vi "Calculate Gains.vi"(1 "DSA Averages":T5, 2 "WT1800 Averages":T3 {"Vrms" format="%.3f"; "Irms" format="%.3f"; "Power" format="%.3f"; "Vpkpk" format="%.3f"; "Ipkpk" format="%.3f"}, 11 "error in":errorcluster, 12 "Error or Abort":bool, 13 "Settings Cluster":T7={"Supply Voltage [Vdc]"=0.0, "Max Supply Current [Idc]"=0.0, "Settling Delay"=0.0, "Temp Criteria"=0.0, "Voltage Steps [Vrms]"=[], "User Notes"="", "Config Wave File Path"=path "", "Config Voltage [Vrms]"=0.0, "Channel Configuration List"={"Channel Configuration Cluster"={"Input"=enum."---", "Enable"=FALSE, "User Notes"="", "Voltage Range"=15.0, "Current Range"=2.5}, "Channel Configuration Cluster 2"={"Input"=enum."---", "Enable"=FALSE, "User Notes"="", "Voltage Range"=15.0, "Current Range"=2.5}, "Channel Configuration Cluster 3"={"Input"=enum."---", "Enable"=FALSE, "User Notes"="", "Voltage Range"=15.0, "Current Range"=2.5}, "Channel Configuration Cluster 4"={"Input"=enum."---", "Enable"=FALSE, "User Notes"="", "Voltage Range"=15.0, "Current Range"=2.5}, "Channel Configuration Cluster 5"={"Input"=enum."---", "Enable"=FALSE, "User Notes"="", "Voltage Range"=15.0, "Current Range"=2.5}, "Channel Configuration Cluster 6"={"Input"=enum."---", "Enable"=FALSE, "User Notes"="", "Voltage Range"=15.0, "Current Range"=2.5}, "Channel Configuration Cluster 7"={"Input"=enum."---", "Enable"=FALSE, "User Notes"="", "Voltage Range"=15.0, "Current Range"=2.5}, "Channel Configuration Cluster 8"={"Input"=enum."---", "Enable"=FALSE, "User Notes"="", "Voltage Range"=15.0, "Current Range"=2.5}, "Channel Configuration Cluster 9"={"Input"=enum."---", "Enable"=FALSE, "User Notes"="", "Voltage Range"=15.0, "Current Range"=2.5}, "Channel Configuration Cluster 10"={"Input"=enum."---", "Enable"=FALSE, "User Notes"="", "Voltage Range"=15.0, "Current Range"=25.0}, "Channel Configuration Cluster 11"={"Input"=enum."---", "Enable"=FALSE, "User Notes"="", "Voltage Range"=15.0, "Current Range"=25.0}, "Channel Configuration Cluster 12"={"Input"=enum."---", "Enable"=FALSE, "User Notes"="", "Voltage Range"=15.0, "Current Range"=25.0}, "Channel Configuration Cluster 13"={"Input"=enum."---", "Enable"=FALSE, "User Notes"="", "Voltage Range"=15.0, "Current Range"=25.0}, "Channel Configuration Cluster 14"={"Input"=enum."---", "Enable"=FALSE, "User Notes"="", "Voltage Range"=15.0, "Current Range"=25.0}, "Channel Configuration Cluster 15"={"Input"=enum."---", "Enable"=FALSE, "User Notes"="", "Voltage Range"=15.0, "Current Range"=25.0}, "Channel Configuration Cluster 16"={"Input"=enum."---", "Enable"=FALSE, "User Notes"="", "Voltage Range"=15.0, "Current Range"=25.0}, "Channel Configuration Cluster 17"={"Input"=enum."---", "Enable"=FALSE, "User Notes"="", "Voltage Range"=15.0, "Current Range"=25.0}}, "User Gains"={"Gain 1"=0.0, "Gain 2"=0.0, "Gain 3"=0.0, "Gain 4"=0.0, "Gain 5"=0.0, "Gain 6"=0.0}, "Gains"={"Gain 1"=0.0, "Gain 2"=0.0, "Gain 3"=0.0, "Gain 4"=0.0, "Gain 5"=0.0, "Gain 6"=0.0}, "Gain Array"={"Gain 1"=0.0, "Gain 2"=0.0, "Gain 3"=0.0, "Gain 4"=0.0, "Gain 5"=0.0, "Gain 6"=0.0, "Gain 7"=0.0, "Gain 8"=0.0, "Gain 9"=0.0, "Gain 10"=0.0, "Gain 11"=0.0, "Gain 12"=0.0, "Gain 13"=0.0, "Gain 14"=0.0, "Gain 15"=0.0, "Gain 16"=0.0, "Gain 17"=0.0}, "Wave File Path 1"=path "", "Wave File Path 2"=path "", "Wave File Path 3"=path "", "Wave File Path 4"=path "", "Range"=FALSE, "CF"=FALSE} {"Gain Array"."Gain 17" format="%.2f"; "Gain Array"."Gain 16" format="%.2f"; "Gain Array"."Gain 15" format="%.2f"; "Gain Array"."Gain 14" format="%.2f"; "Gain Array"."Gain 13" format="%.2f"; "Gain Array"."Gain 12" format="%.2f"; "Gain Array"."Gain 11" format="%.2f"; "Gain Array"."Gain 10" format="%.2f"; "Gain Array"."Gain 9" format="%.2f"; "Gain Array"."Gain 8" format="%.2f"; "Gain Array"."Gain 7" format="%.2f"; "Gain Array"."Gain 6" format="%.2f"; "Gain Array"."Gain 5" format="%.2f"; "Gain Array"."Gain 4" format="%.2f"; "Gain Array"."Gain 3" format="%.2f"; "Gain Array"."Gain 2" format="%.2f"; "Gain Array"."Gain 1" format="%.2f"; "Gains"."Gain 6" format="%.2f"; "Gains"."Gain 5" format="%.2f"; "Gains"."Gain 4" format="%.2f"; "Gains"."Gain 3" format="%.2f"; "Gains"."Gain 2" format="%.2f"; "Gains"."Gain 1" format="%.2f"; "User Gains"."Gain 6" format="%.2f"; "User Gains"."Gain 5" format="%.2f"; "User Gains"."Gain 4" format="%.2f"; "User Gains"."Gain 3" format="%.2f"; "User Gains"."Gain 2" format="%.2f"; "User Gains"."Gain 1" format="%.2f"; "Channel Configuration List"."Channel Configuration Cluster 17"."Current Range" items=["1 <500m>"=0.5, "2 <1>"=1.0, "5 <2.5>"=2.5, "10 <5>"=5.0, "20 <10>"=10.0, "50 <25>"=25.0]; "Channel Configuration List"."Channel Configuration Cluster 17"."Voltage Range" items=["1.5 <0.75>"=0.75, "3 <1.5>"=1.5, "6 <3>"=3.0, "10 <5>"=5.0, "15 <7.5>"=7.5, "30 <15>"=15.0, "60 <30>"=30.0, "100 <50>"=50.0, "150 <75>"=75.0, "300 <150>"=150.0, "600 <300>"=300.0, "1000 <500>"=500.0]; "Channel Configuration List"."Channel Configuration Cluster 16"."Current Range" items=["1 <500m>"=0.5, "2 <1>"=1.0, "5 <2.5>"=2.5, "10 <5>"=5.0, "20 <10>"=10.0, "50 <25>"=25.0]; "Channel Configuration List"."Channel Configuration Cluster 16"."Voltage Range" items=["1.5 <0.75>"=0.75, "3 <1.5>"=1.5, "6 <3>"=3.0, "10 <5>"=5.0, "15 <7.5>"=7.5, "30 <15>"=15.0, "60 <30>"=30.0, "100 <50>"=50.0, "150 <75>"=75.0, "300 <150>"=150.0, "600 <300>"=300.0, "1000 <500>"=500.0]; "Channel Configuration List"."Channel Configuration Cluster 15"."Current Range" items=["1 <500m>"=0.5, "2 <1>"=1.0, "5 <2.5>"=2.5, "10 <5>"=5.0, "20 <10>"=10.0, "50 <25>"=25.0]; "Channel Configuration List"."Channel Configuration Cluster 15"."Voltage Range" items=["1.5 <0.75>"=0.75, "3 <1.5>"=1.5, "6 <3>"=3.0, "10 <5>"=5.0, "15 <7.5>"=7.5, "30 <15>"=15.0, "60 <30>"=30.0, "100 <50>"=50.0, "150 <75>"=75.0, "300 <150>"=150.0, "600 <300>"=300.0, "1000 <500>"=500.0]; "Channel Configuration List"."Channel Configuration Cluster 14"."Current Range" items=["1 <500m>"=0.5, "2 <1>"=1.0, "5 <2.5>"=2.5, "10 <5>"=5.0, "20 <10>"=10.0, "50 <25>"=25.0]; "Channel Configuration List"."Channel Configuration Cluster 14"."Voltage Range" items=["1.5 <0.75>"=0.75, "3 <1.5>"=1.5, "6 <3>"=3.0, "10 <5>"=5.0, "15 <7.5>"=7.5, "30 <15>"=15.0, "60 <30>"=30.0, "100 <50>"=50.0, "150 <75>"=75.0, "300 <150>"=150.0, "600 <300>"=300.0, "1000 <500>"=500.0]; "Channel Configuration List"."Channel Configuration Cluster 13"."Current Range" items=["1 <500m>"=0.5, "2 <1>"=1.0, "5 <2.5>"=2.5, "10 <5>"=5.0, "20 <10>"=10.0, "50 <25>"=25.0]; "Channel Configuration List"."Channel Configuration Cluster 13"."Voltage Range" items=["1.5 <0.75>"=0.75, "3 <1.5>"=1.5, "6 <3>"=3.0, "10 <5>"=5.0, "15 <7.5>"=7.5, "30 <15>"=15.0, "60 <30>"=30.0, "100 <50>"=50.0, "150 <75>"=75.0, "300 <150>"=150.0, "600 <300>"=300.0, "1000 <500>"=500.0]; "Channel Configuration List"."Channel Configuration Cluster 12"."Current Range" items=["1 <500m>"=0.5, "2 <1>"=1.0, "5 <2.5>"=2.5, "10 <5>"=5.0, "20 <10>"=10.0, "50 <25>"=25.0]; "Channel Configuration List"."Channel Configuration Cluster 12"."Voltage Range" items=["1.5 <0.75>"=0.75, "3 <1.5>"=1.5, "6 <3>"=3.0, "10 <5>"=5.0, "15 <7.5>"=7.5, "30 <15>"=15.0, "60 <30>"=30.0, "100 <50>"=50.0, "150 <75>"=75.0, "300 <150>"=150.0, "600 <300>"=300.0, "1000 <500>"=500.0]; "Channel Configuration List"."Channel Configuration Cluster 11"."Current Range" items=["1 <500m>"=0.5, "2 <1>"=1.0, "5 <2.5>"=2.5, "10 <5>"=5.0, "20 <10>"=10.0, "50 <25>"=25.0]; "Channel Configuration List"."Channel Configuration Cluster 11"."Voltage Range" items=["1.5 <0.75>"=0.75, "3 <1.5>"=1.5, "6 <3>"=3.0, "10 <5>"=5.0, "15 <7.5>"=7.5, "30 <15>"=15.0, "60 <30>"=30.0, "100 <50>"=50.0, "150 <75>"=75.0, "300 <150>"=150.0, "600 <300>"=300.0, "1000 <500>"=500.0]; "Channel Configuration List"."Channel Configuration Cluster 10"."Current Range" items=["1 <500m>"=0.5, "2 <1>"=1.0, "5 <2.5>"=2.5, "10 <5>"=5.0, "20 <10>"=10.0, "50 <25>"=25.0]; "Channel Configuration List"."Channel Configuration Cluster 10"."Voltage Range" items=["1.5 <0.75>"=0.75, "3 <1.5>"=1.5, "6 <3>"=3.0, "10 <5>"=5.0, "15 <7.5>"=7.5, "30 <15>"=15.0, "60 <30>"=30.0, "100 <50>"=50.0, "150 <75>"=75.0, "300 <150>"=150.0, "600 <300>"=300.0, "1000 <500>"=500.0]; "Channel Configuration List"."Channel Configuration Cluster 9"."Voltage Range" items=["1.5 <0.75>"=0.75, "3 <1.5>"=1.5, "6 <3>"=3.0, "10 <5>"=5.0, "15 <7.5>"=7.5, "30 <15>"=15.0, "60 <30>"=30.0, "100 <50>"=50.0, "150 <75>"=75.0, "300 <150>"=150.0, "600 <300>"=300.0, "1000 <500>"=500.0]; "Channel Configuration List"."Channel Configuration Cluster 9"."Current Range" items=["10m <5m>"=0.005, "20m <10m>"=0.01, "50m <25m>"=0.025, "100m <50m>"=0.05, "200m <100m>"=0.1, "500m <250m>"=0.25, "1 <500m>"=0.5, "2 <1>"=1.0, "5 <2.5>"=2.5]; "Channel Configuration List"."Channel Configuration Cluster 8"."Voltage Range" items=["1.5 <0.75>"=0.75, "3 <1.5>"=1.5, "6 <3>"=3.0, "10 <5>"=5.0, "15 <7.5>"=7.5, "30 <15>"=15.0, "60 <30>"=30.0, "100 <50>"=50.0, "150 <75>"=75.0, "300 <150>"=150.0, "600 <300>"=300.0, "1000 <500>"=500.0]; "Channel Configuration List"."Channel Configuration Cluster 8"."Current Range" items=["10m <5m>"=0.005, "20m <10m>"=0.01, "50m <25m>"=0.025, "100m <50m>"=0.05, "200m <100m>"=0.1, "500m <250m>"=0.25, "1 <500m>"=0.5, "2 <1>"=1.0, "5 <2.5>"=2.5]; "Channel Configuration List"."Channel Configuration Cluster 7"."Voltage Range" items=["1.5 <0.75>"=0.75, "3 <1.5>"=1.5, "6 <3>"=3.0, "10 <5>"=5.0, "15 <7.5>"=7.5, "30 <15>"=15.0, "60 <30>"=30.0, "100 <50>"=50.0, "150 <75>"=75.0, "300 <150>"=150.0, "600 <300>"=300.0, "1000 <500>"=500.0]; "Channel Configuration List"."Channel Configuration Cluster 7"."Current Range" items=["10m <5m>"=0.005, "20m <10m>"=0.01, "50m <25m>"=0.025, "100m <50m>"=0.05, "200m <100m>"=0.1, "500m <250m>"=0.25, "1 <500m>"=0.5, "2 <1>"=1.0, "5 <2.5>"=2.5]; "Channel Configuration List"."Channel Configuration Cluster 6"."Voltage Range" items=["1.5 <0.75>"=0.75, "3 <1.5>"=1.5, "6 <3>"=3.0, "10 <5>"=5.0, "15 <7.5>"=7.5, "30 <15>"=15.0, "60 <30>"=30.0, "100 <50>"=50.0, "150 <75>"=75.0, "300 <150>"=150.0, "600 <300>"=300.0, "1000 <500>"=500.0]; "Channel Configuration List"."Channel Configuration Cluster 6"."Current Range" items=["10m <5m>"=0.005, "20m <10m>"=0.01, "50m <25m>"=0.025, "100m <50m>"=0.05, "200m <100m>"=0.1, "500m <250m>"=0.25, "1 <500m>"=0.5, "2 <1>"=1.0, "5 <2.5>"=2.5]; "Channel Configuration List"."Channel Configuration Cluster 5"."Voltage Range" items=["1.5 <0.75>"=0.75, "3 <1.5>"=1.5, "6 <3>"=3.0, "10 <5>"=5.0, "15 <7.5>"=7.5, "30 <15>"=15.0, "60 <30>"=30.0, "100 <50>"=50.0, "150 <75>"=75.0, "300 <150>"=150.0, "600 <300>"=300.0, "1000 <500>"=500.0]; "Channel Configuration List"."Channel Configuration Cluster 5"."Current Range" items=["10m <5m>"=0.005, "20m <10m>"=0.01, "50m <25m>"=0.025, "100m <50m>"=0.05, "200m <100m>"=0.1, "500m <250m>"=0.25, "1 <500m>"=0.5, "2 <1>"=1.0, "5 <2.5>"=2.5]; "Channel Configuration List"."Channel Configuration Cluster 4"."Voltage Range" items=["1.5 <0.75>"=0.75, "3 <1.5>"=1.5, "6 <3>"=3.0, "10 <5>"=5.0, "15 <7.5>"=7.5, "30 <15>"=15.0, "60 <30>"=30.0, "100 <50>"=50.0, "150 <75>"=75.0, "300 <150>"=150.0, "600 <300>"=300.0, "1000 <500>"=500.0]; "Channel Configuration List"."Channel Configuration Cluster 4"."Current Range" items=["10m <5m>"=0.005, "20m <10m>"=0.01, "50m <25m>"=0.025, "100m <50m>"=0.05, "200m <100m>"=0.1, "500m <250m>"=0.25, "1 <500m>"=0.5, "2 <1>"=1.0, "5 <2.5>"=2.5]; "Channel Configuration List"."Channel Configuration Cluster 3"."Voltage Range" items=["1.5 <0.75>"=0.75, "3 <1.5>"=1.5, "6 <3>"=3.0, "10 <5>"=5.0, "15 <7.5>"=7.5, "30 <15>"=15.0, "60 <30>"=30.0, "100 <50>"=50.0, "150 <75>"=75.0, "300 <150>"=150.0, "600 <300>"=300.0, "1000 <500>"=500.0]; "Channel Configuration List"."Channel Configuration Cluster 3"."Current Range" items=["10m <5m>"=0.005, "20m <10m>"=0.01, "50m <25m>"=0.025, "100m <50m>"=0.05, "200m <100m>"=0.1, "500m <250m>"=0.25, "1 <500m>"=0.5, "2 <1>"=1.0, "5 <2.5>"=2.5]; "Channel Configuration List"."Channel Configuration Cluster 2"."Voltage Range" items=["1.5 <0.75>"=0.75, "3 <1.5>"=1.5, "6 <3>"=3.0, "10 <5>"=5.0, "15 <7.5>"=7.5, "30 <15>"=15.0, "60 <30>"=30.0, "100 <50>"=50.0, "150 <75>"=75.0, "300 <150>"=150.0, "600 <300>"=300.0, "1000 <500>"=500.0]; "Channel Configuration List"."Channel Configuration Cluster 2"."Current Range" items=["10m <5m>"=0.005, "20m <10m>"=0.01, "50m <25m>"=0.025, "100m <50m>"=0.05, "200m <100m>"=0.1, "500m <250m>"=0.25, "1 <500m>"=0.5, "2 <1>"=1.0, "5 <2.5>"=2.5]; "Channel Configuration List"."Channel Configuration Cluster"."Voltage Range" items=["1.5 <0.75>"=0.75, "3 <1.5>"=1.5, "6 <3>"=3.0, "10 <5>"=5.0, "15 <7.5>"=7.5, "30 <15>"=15.0, "60 <30>"=30.0, "100 <50>"=50.0, "150 <75>"=75.0, "300 <150>"=150.0, "600 <300>"=300.0, "1000 <500>"=500.0]; "Channel Configuration List"."Channel Configuration Cluster"."Current Range" items=["10m <5m>"=0.005, "20m <10m>"=0.01, "50m <25m>"=0.025, "100m <50m>"=0.05, "200m <100m>"=0.1, "500m <250m>"=0.25, "1 <500m>"=0.5, "2 <1>"=1.0, "5 <2.5>"=2.5]; "Settling Delay" min=0.0 format="%<%H:%M:%S>t"}) -> (4 "Average Power":sgl[](array[numeric]) format="%.3g", 6 "Gain Averages":T1 {"Gain 6" format="%.2f"; "Gain 5" format="%.2f"; "Gain 4" format="%.2f"; "Gain 3" format="%.2f"; "Gain 2" format="%.2f"; "Gain 1" format="%.2f"}, 8 "Gain Array":T2 {"Gain 17" format="%.2f"; "Gain 16" format="%.2f"; "Gain 15" format="%.2f"; "Gain 14" format="%.2f"; "Gain 13" format="%.2f"; "Gain 12" format="%.2f"; "Gain 11" format="%.2f"; "Gain 10" format="%.2f"; "Gain 9" format="%.2f"; "Gain 8" format="%.2f"; "Gain 7" format="%.2f"; "Gain 6" format="%.2f"; "Gain 5" format="%.2f"; "Gain 4" format="%.2f"; "Gain 3" format="%.2f"; "Gain 2" format="%.2f"; "Gain 1" format="%.2f"}, 14 "Impedances":dbl[](array[numeric]) format="%.3g", 15 "error out":errorcluster)   [LabVIEW 2021]
uses:
  Controls/Settings Control.ctl
  Controls/Channel Configuration List.ctl
  Controls/Channel Configuration Cluster.ctl
  Controls/Channel Configuration Cluster High Current.ctl
  Controls/Gain Averages.ctl
  Controls/Gain Array.ctl
  Controls/WT1800 Measurements.ctl
  Controls/WT1800 Readings.ctl
  Controls/DSA Measurements.ctl
  Controls/DSA Readings.ctl
  <vilib>/Analysis/baseanly.llb/Mean (DBL).vi
  <vilib>/Analysis/NI_AALBase.lvlib
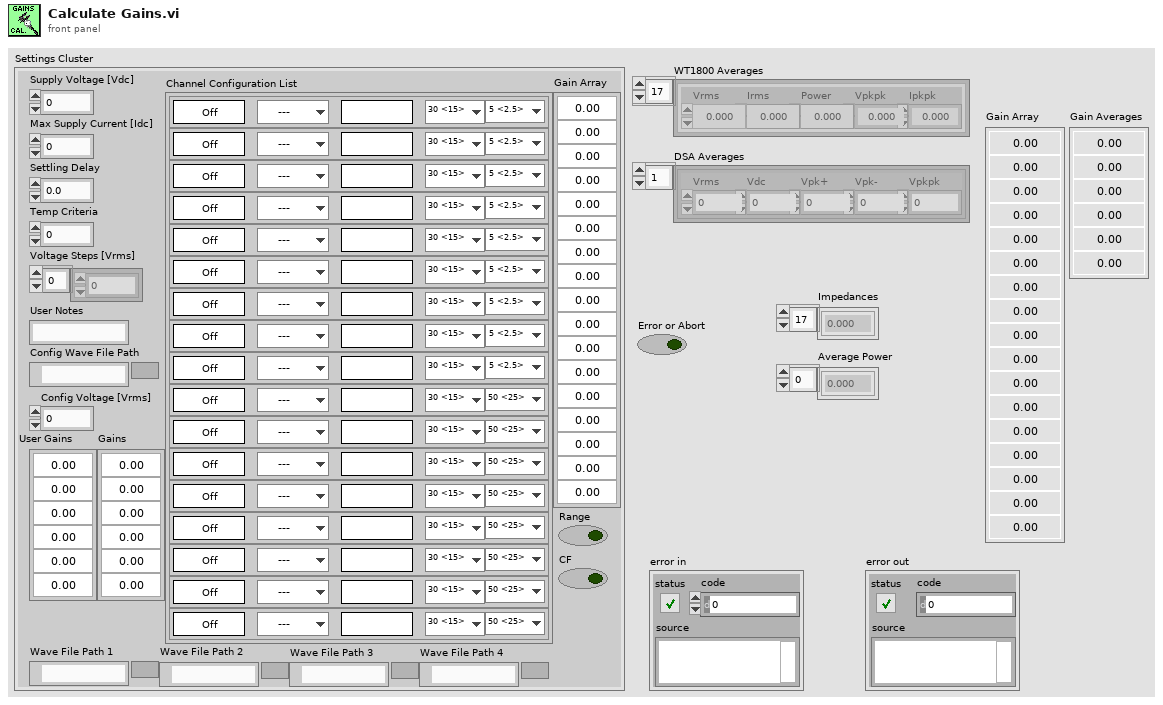
[diagram p1: front panel]
types:
  T1 = typedef "Gain Averages.ctl" = cluster{"Gain 1":dbl, "Gain 2":dbl, "Gain 3":dbl, "Gain 4":dbl, "Gain 5":dbl, "Gain 6":dbl}
  T2 = typedef "Gain Array.ctl" = cluster{"Gain 1":dbl, "Gain 2":dbl, "Gain 3":dbl, "Gain 4":dbl, "Gain 5":dbl, "Gain 6":dbl, "Gain 7":dbl, "Gain 8":dbl, "Gain 9":dbl, "Gain 10":dbl, "Gain 11":dbl, "Gain 12":dbl, "Gain 13":dbl, "Gain 14":dbl, "Gain 15":dbl, "Gain 16":dbl, "Gain 17":dbl}
  T3 = typedef "WT1800 Measurements.ctl" = T4[]
  T4 = typedef "WT1800 Readings.ctl" = cluster{"Vrms":sgl, "Irms":sgl, "Power":sgl, "Vpkpk":sgl, "Ipkpk":sgl}
  T5 = typedef "DSA Measurements.ctl" = T6[]
  T6 = typedef "DSA Readings.ctl" = cluster{"Vrms":sgl, "Vdc":sgl, "Vpk+":sgl, "Vpk-":sgl, "Vpkpk":sgl}
  T7 = typedef "Settings Control.ctl" = cluster{"Supply Voltage [Vdc]":sgl, "Max Supply Current [Idc]":sgl, "Settling Delay":dbl, "Temp Criteria":sgl, "Voltage Steps [Vrms]":sgl[], "User Notes":string, "Config Wave File Path":path, "Config Voltage [Vrms]":sgl, "Channel Configuration List":T8, "User Gains":T1, "Gains":T1, "Gain Array":T2, "Wave File Path 1":path, "Wave File Path 2":path, "Wave File Path 3":path, "Wave File Path 4":path, "Range":bool, "CF":bool}
  T8 = typedef "Channel Configuration List.ctl" = cluster{"Channel Configuration Cluster":T9, "Channel Configuration Cluster 2":T9, "Channel Configuration Cluster 3":T9, "Channel Configuration Cluster 4":T9, "Channel Configuration Cluster 5":T9, "Channel Configuration Cluster 6":T9, "Channel Configuration Cluster 7":T9, "Channel Configuration Cluster 8":T9, "Channel Configuration Cluster 9":T9, "Channel Configuration Cluster 10":T10, "Channel Configuration Cluster 11":T10, "Channel Configuration Cluster 12":T10, "Channel Configuration Cluster 13":T10, "Channel Configuration Cluster 14":T10, "Channel Configuration Cluster 15":T10, "Channel Configuration Cluster 16":T10, "Channel Configuration Cluster 17":T10}
  T9 = typedef "Channel Configuration Cluster.ctl" = cluster{"Input":enum16{"---", "1", "1 AVG", "2", "2 AVG", "3", "3 AVG", "4", "4 AVG"}, "Enable":bool, "User Notes":string, "Voltage Range":dbl, "Current Range":dbl}
  T10 = typedef "Channel Configuration Cluster High Current.ctl" = cluster{"Input":enum16{"---", "1", "1 AVG", "2", "2 AVG", "3", "3 AVG", "4", "4 AVG"}, "Enable":bool, "User Notes":string, "Voltage Range":dbl, "Current Range":dbl}
  T11 = enum16{"---", "1", "1 AVG", "2", "2 AVG", "3", "3 AVG", "4", "4 AVG"}
  T12 = cluster{"[0]":dbl, "[1]":dbl, "[2]":dbl, "[3]":dbl, "[4]":dbl, "[5]":dbl}
  T13 = cluster{"[0]":dbl, "[1]":dbl, "[2]":dbl, "[3]":dbl, "[4]":dbl, "[5]":dbl, "[6]":dbl, "[7]":dbl, "[8]":dbl, "[9]":dbl, "[10]":dbl, "[11]":dbl, "[12]":dbl, "[13]":dbl, "[14]":dbl, "[15]":dbl, "[16]":dbl}
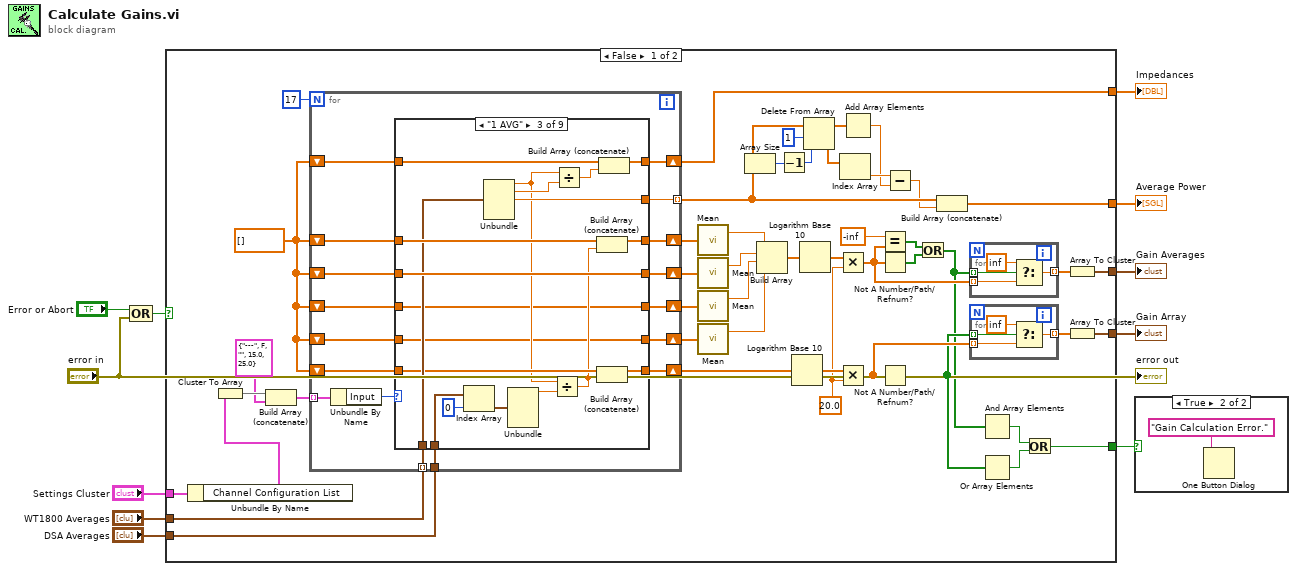
[diagram p0: block diagram]
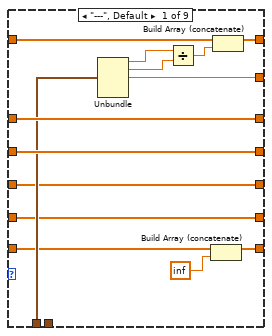
[diagram p3: hidden frame]
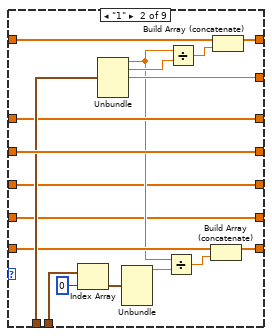
[diagram p4: hidden frame]
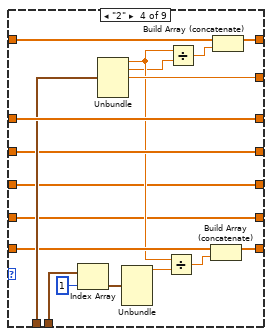
[diagram p5: hidden frame]
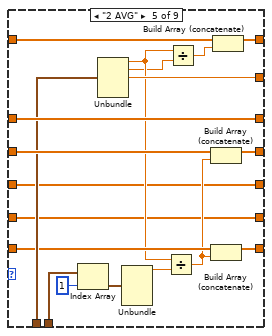
[diagram p6: hidden frame]
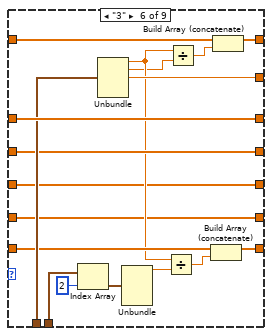
[diagram p7: hidden frame]
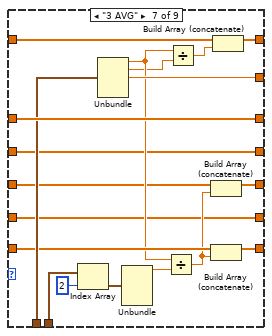
[diagram p8: hidden frame]
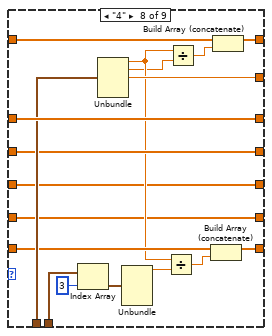
[diagram p9: hidden frame]
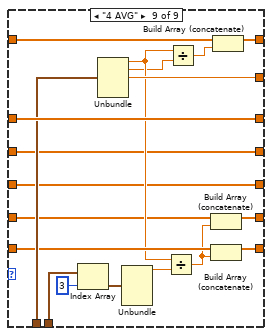
[diagram p10: hidden frame]
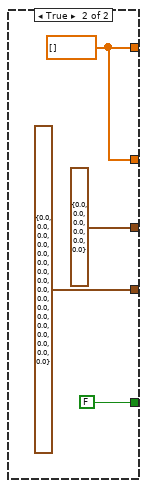
[diagram p11: hidden frame]
diagram:
  n1 = Compound Arithmetic op=OR("Error or Abort", "error in") -> (w4:bool)
  n2 = case shown="False" w4 {
    tunnel: "Settings Cluster" -> [w38 _]
    tunnel: "DSA Averages" -> [w36 _]
    tunnel: "WT1800 Averages" -> [w37 _]
    tunnel: [w35 w249] -> w11
    tunnel: [w56 T2 {"Gain 1"=0.0, "Gain 2"=0.0, "Gain 3"=0.0, "Gain 4"=0.0, "Gain 5"=0.0, "Gain 6"=0.0, "Gain 7"=0.0, "Gain 8"=0.0, "Gain 9"=0.0, "Gain 10"=0.0, "Gain 11"=0.0, "Gain 12"=0.0, "Gain 13"=0.0, "Gain 14"=0.0, "Gain 15"=0.0, "Gain 16"=0.0, "Gain 17"=0.0} ("Gain Array")] -> w9
    tunnel: [w53 T1 {"Gain 1"=0.0, "Gain 2"=0.0, "Gain 3"=0.0, "Gain 4"=0.0, "Gain 5"=0.0, "Gain 6"=0.0} ("Gain Averages")] -> w10
    tunnel: [w34 w249] -> w2
    tunnel: [w33 FALSE] -> w1
    frame False {
      w50 = 20.0
      w17 = dbl[] [] ("Gains for Ch1")
      n3 = Unbundle By Name(w38) -> ("Channel Configuration List"=w13:T8)
      n4 = Cluster To Array(cluster=w13) -> (array=w49:T10[])
      n5 = Build Array (concatenate)(w49, T10 {"Input"=enum."---", "Enable"=FALSE, "User Notes"="", "Voltage Range"=15.0, "Current Range"=25.0} ("Channel Configuration Cluster")) -> (w39:T10[])
      n6 = for {
        N: 17 -> [_]
        tunnel: w39 -> [w76] mode=indexing
        tunnel: w36 -> [w83]
        tunnel: w37 -> [w82] mode=indexing
        tunnel: [w81] -> w47 mode=indexing
        shift-right: [w80] -> w58
        shift-left: w17 -> [w79]
        shift-right: [w77] -> w57
        shift-left: w17 -> [w78]
        shift-right: [w74] -> w30
        shift-left: w17 -> [w73]
        shift-right: [w71] -> w34
        shift-left: w17 -> [w72]
        shift-right: [w69] -> w18
        shift-left: w17 -> [w70]
        shift-right: [w67] -> w19
        shift-left: w17 -> [w68]
        n7 = Unbundle By Name(w76) -> ("Input"=w75:T11)
        n8 = case shown="\"1 AVG\"" w75 {
          tunnel: w83 -> [_ w113 w132 w150 w169 w187 w206 w224 w243]
          tunnel: w82 -> [w94 w109 w126 w146 w164 w183 w202 w220 w239]
          tunnel: [w96 w108 w129 w147 w165 w184 w203 w221 w240] -> w80
          tunnel: [w97 w112 w131 w149 w168 w186 w205 w223 w242] -> w81
          tunnel: w79 -> [w96 w108 w128 w147 w165 w184 w203 w221 w240]
          tunnel: [w95 w110 w127 w145 w163 w182 w191 w219 w227] -> w77
          tunnel: w78 -> [w95 w110 w127 w145 w166 w182 w191 w219 w227]
          tunnel: [w92 w106 w124 w143 w161 w180 w200 w217 w237] -> w74
          tunnel: w73 -> [w93 w105 w125 w144 w162 w181 w201 w218 w238]
          tunnel: w72 -> [w87 w101 w119 w138 w156 w175 w195 w212 w232]
          tunnel: [w86 w100 w118 w137 w155 w174 w194 w211 w231] -> w71
          tunnel: w70 -> [w85 w99 w117 w136 w154 w173 w193 w210 w230]
          tunnel: [w85 w99 w117 w136 w154 w173 w192 w210 w230] -> w69
          tunnel: w68 -> [w84 w98 w116 w135 w153 w172 w190 w209 w229]
          tunnel: [w84 w98 w116 w135 w153 w172 w190 w209 w228] -> w67
          frame "---", Default {
            n9 = Unbundle(w94) -> ("Vrms"=w88:sgl, "Irms"=w89:sgl, "Power"=w97:sgl)  [unwired: 2 out]
            n10 = Divide(x=w88, y=w89) -> (x/y=w90:sgl)
            n11 = Build Array (concatenate)(w93, inf) -> (w92:dbl[])
            n12 = Build Array (concatenate)(w87, w90) -> (w86:dbl[])
          }
          frame "1" {
            n13 = Index Array(array=w113, index=0) -> (element=w114:T6)
            n14 = Unbundle(w109) -> ("Vrms"=w102:sgl, "Irms"=w103:sgl, "Power"=w112:sgl)  [unwired: 2 out]
            n15 = Unbundle(w114) -> ("Vrms"=w115:sgl)  [unwired: 4 out]
            n16 = Divide(x=w102, y=w115) -> (x/y=w107:sgl)
            n17 = Divide(x=w102, y=w103) -> (x/y=w104:sgl)
            n18 = Build Array (concatenate)(w105, w107) -> (w106:dbl[])
            n19 = Build Array (concatenate)(w101, w104) -> (w100:dbl[])
          }
          frame "1 AVG" {
            n20 = Index Array(array=w132, index=0) -> (element=w133:T6)
            n21 = Unbundle(w126) -> ("Vrms"=w120:sgl, "Irms"=w121:sgl, "Power"=w131:sgl)  [unwired: 2 out]
            n22 = Unbundle(w133) -> ("Vrms"=w134:sgl)  [unwired: 4 out]
            n23 = Divide(x=w120, y=w134) -> (x/y=w123:sgl)
            n24 = Divide(x=w120, y=w121) -> (x/y=w122:sgl)
            n25 = Build Array (concatenate)(w128, w123) -> (w129:dbl[])
            n26 = Build Array (concatenate)(w125, w123) -> (w124:dbl[])
            n27 = Build Array (concatenate)(w119, w122) -> (w118:dbl[])
          }
          frame "2" {
            n28 = Index Array(array=w150, index=1) -> (element=w151:T6)
            n29 = Unbundle(w146) -> ("Vrms"=w140:sgl, "Irms"=w139:sgl, "Power"=w149:sgl)  [unwired: 2 out]
            n30 = Unbundle(w151) -> ("Vrms"=w152:sgl)  [unwired: 4 out]
            n31 = Divide(x=w140, y=w152) -> (x/y=w142:sgl)
            n32 = Divide(x=w140, y=w139) -> (x/y=w141:sgl)
            n33 = Build Array (concatenate)(w144, w142) -> (w143:dbl[])
            n34 = Build Array (concatenate)(w138, w141) -> (w137:dbl[])
          }
          frame "2 AVG" {
            n35 = Index Array(array=w169, index=1) -> (element=w170:T6)
            n36 = Unbundle(w164) -> ("Vrms"=w158:sgl, "Irms"=w157:sgl, "Power"=w168:sgl)  [unwired: 2 out]
            n37 = Unbundle(w170) -> ("Vrms"=w171:sgl)  [unwired: 4 out]
            n38 = Divide(x=w158, y=w171) -> (x/y=w160:sgl)
            n39 = Divide(x=w158, y=w157) -> (x/y=w159:sgl)
            n40 = Build Array (concatenate)(w166, w160) -> (w163:dbl[])
            n41 = Build Array (concatenate)(w162, w160) -> (w161:dbl[])
            n42 = Build Array (concatenate)(w156, w159) -> (w155:dbl[])
          }
          frame "3" {
            n43 = Index Array(array=w187, index=2) -> (element=w188:T6)
            n44 = Unbundle(w183) -> ("Vrms"=w177:sgl, "Irms"=w176:sgl, "Power"=w186:sgl)  [unwired: 2 out]
            n45 = Unbundle(w188) -> ("Vrms"=w189:sgl)  [unwired: 4 out]
            n46 = Divide(x=w177, y=w189) -> (x/y=w179:sgl)
            n47 = Divide(x=w177, y=w176) -> (x/y=w178:sgl)
            n48 = Build Array (concatenate)(w181, w179) -> (w180:dbl[])
            n49 = Build Array (concatenate)(w175, w178) -> (w174:dbl[])
          }
          frame "3 AVG" {
            n50 = Index Array(array=w206, index=2) -> (element=w207:T6)
            n51 = Unbundle(w202) -> ("Vrms"=w197:sgl, "Irms"=w196:sgl, "Power"=w205:sgl)  [unwired: 2 out]
            n52 = Unbundle(w207) -> ("Vrms"=w208:sgl)  [unwired: 4 out]
            n53 = Divide(x=w197, y=w208) -> (x/y=w199:sgl)
            n54 = Divide(x=w197, y=w196) -> (x/y=w198:sgl)
            n55 = Build Array (concatenate)(w193, w199) -> (w192:dbl[])
            n56 = Build Array (concatenate)(w201, w199) -> (w200:dbl[])
            n57 = Build Array (concatenate)(w195, w198) -> (w194:dbl[])
          }
          frame "4" {
            n58 = Index Array(array=w224, index=3) -> (element=w225:T6)
            n59 = Unbundle(w220) -> ("Vrms"=w214:sgl, "Irms"=w213:sgl, "Power"=w223:sgl)  [unwired: 2 out]
            n60 = Unbundle(w225) -> ("Vrms"=w226:sgl)  [unwired: 4 out]
            n61 = Divide(x=w214, y=w226) -> (x/y=w216:sgl)
            n62 = Divide(x=w214, y=w213) -> (x/y=w215:sgl)
            n63 = Build Array (concatenate)(w218, w216) -> (w217:dbl[])
            n64 = Build Array (concatenate)(w212, w215) -> (w211:dbl[])
          }
          frame "4 AVG" {
            n65 = Index Array(array=w243, index=3) -> (element=w244:T6)
            n66 = Unbundle(w239) -> ("Vrms"=w234:sgl, "Irms"=w233:sgl, "Power"=w242:sgl)  [unwired: 2 out]
            n67 = Unbundle(w244) -> ("Vrms"=w245:sgl)  [unwired: 4 out]
            n68 = Divide(x=w234, y=w245) -> (x/y=w236:sgl)
            n69 = Divide(x=w234, y=w233) -> (x/y=w235:sgl)
            n70 = Build Array (concatenate)(w229, w236) -> (w228:dbl[])
            n71 = Build Array (concatenate)(w238, w236) -> (w237:dbl[])
            n72 = Build Array (concatenate)(w232, w235) -> (w231:dbl[])
          }
        }
      }
      n73 = call-poly <vilib>:"Mean.vi"("X"=w58) -> ("mean"=w55:dbl)  [unwired: 1 out]
      n74 = call-poly <vilib>:"Mean.vi"("X"=w57) -> ("mean"=w14:dbl)  [unwired: 1 out]
      n75 = call-poly <vilib>:"Mean.vi"("X"=w18) -> ("mean"=w15:dbl)  [unwired: 1 out]
      n76 = call-poly <vilib>:"Mean.vi"("X"=w19) -> ("mean"=w16:dbl)  [unwired: 1 out]
      n77 = Array Size(array=w47) -> (size(s)=w45:i32)
      n78 = Build Array(w55, w14, w15, w16) -> (w54:dbl[])
      n79 = Decrement(x=w45) -> (x-1=w44:i32)
      n80 = Logarithm Base 10(1:w30) -> (0:w51:dbl[])
      n81 = Logarithm Base 10(1:w54) -> (0:w52:dbl[])
      n82 = Delete From Array(array=w47, length=1, index=w44) -> (deleted portion=w43:sgl[], array with subset deleted=w46:sgl[])
      n83 = Multiply(x=w52, y=w50) -> (x*y=w23:dbl[])
      n84 = Multiply(x=w51, y=w50) -> (x*y=w27:dbl[])
      n85 = Index Array(array=w43) -> (element=w42:sgl)  [unwired: 1 in]
      n86 = Add Array Elements(numeric array=w46) -> (sum=w41:sgl)
      n87 = Equal?(x=-inf, y=w23) -> (x = y?=w21:bool[])
      n88 = Not A Number/Path/Refnum?(number/path/refnum=w23) -> (NaN/Path/Refnum?=w29:bool[])
      n89 = Not A Number/Path/Refnum?(number/path/refnum=w27) -> (NaN/Path/Refnum?=w25:bool[])
      n90 = Subtract(x=w42, y=w41) -> (x-y=w40:sgl)
      n91 = Or(x=w21, y=w29) -> (x .or. y?=w22:bool[])
      n92 = Build Array (concatenate)(w47, w40) -> (w35:sgl[])
      n93 = for {
        tunnel: w22 -> [w65] mode=indexing
        tunnel: w23 -> [w64] mode=indexing
        tunnel: [w63] -> w28 mode=indexing
        n94 = Select(t=inf, s=w65, f=w64) -> (s? t:f=w63:dbl)
      }
      n95 = for {
        tunnel: w25 -> [w61] mode=indexing
        tunnel: w27 -> [w60] mode=indexing
        tunnel: [w59] -> w26 mode=indexing
        n96 = Select(t=inf, s=w61, f=w60) -> (s? t:f=w59:dbl)
      }
      n97 = And Array Elements(Boolean array=w22) -> (logical AND=w32:bool)
      n98 = Or Array Elements(Boolean array=w25) -> (logical OR=w31:bool)
      n99 = Or(x=w32, y=w31) -> (x .or. y?=w33:bool)
      n100 = Array To Cluster(array=w28) -> (cluster=w53:T12)
      n101 = Array To Cluster(array=w26) -> (cluster=w56:T13)
    }
    frame True {
      w249 = sgl[] []
    }
  }
  "Average Power" <- w11
  "Gain Averages" <- w10
  "Gain Array" <- w9
  "Impedances" <- w2
  n102 = case shown="True" w1 {
    frame False {
    }
    frame True {
      n103 = One Button Dialog(message="Gain Calculation Error.") -> ()  [unwired: 1 in, 1 out]
    }
  }
  "error out" <- "error in"
